vi "BioFLEX Board Switch TEENSY.vi"() -> ()   [LabVIEW 2015]
uses:
  <vilib>/DAQmx/write.llb/DAQmx Write (Digital 1D Bool 1Chan 1Samp).vi
  <vilib>/DAQmx/create/channels.llb/DAQmx Create Channel (DO-Digital Output).vi
  <vilib>/DAQmx/miscellaneous.llb/DAQmx Fill In Error Info.vi
panel:
  in  "MUX 4":T1(ring)
  in  "MUX 3":T1(ring)
  in  "MUX 2":T1(ring)
  in  "MUX 1":T1(ring)
  in  "MUX 4 Enable":bool=TRUE
  in  "MUX 3 Enable":bool=TRUE
  in  "stop":bool
  in  "MUX 1 Enable":bool=TRUE
  in  "MUX 2 Enable":bool=TRUE
  in  "POWER":bool
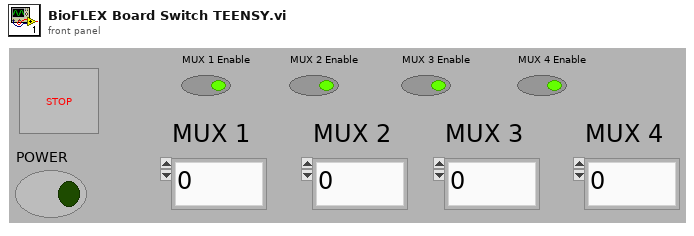
[diagram p1: front panel]
types:
  T1 = enum16{"0", "1", "2", "3", "4", "5", "6", "7", "8", "9", "10", "11", "12", "13", "14", "15", "16"}
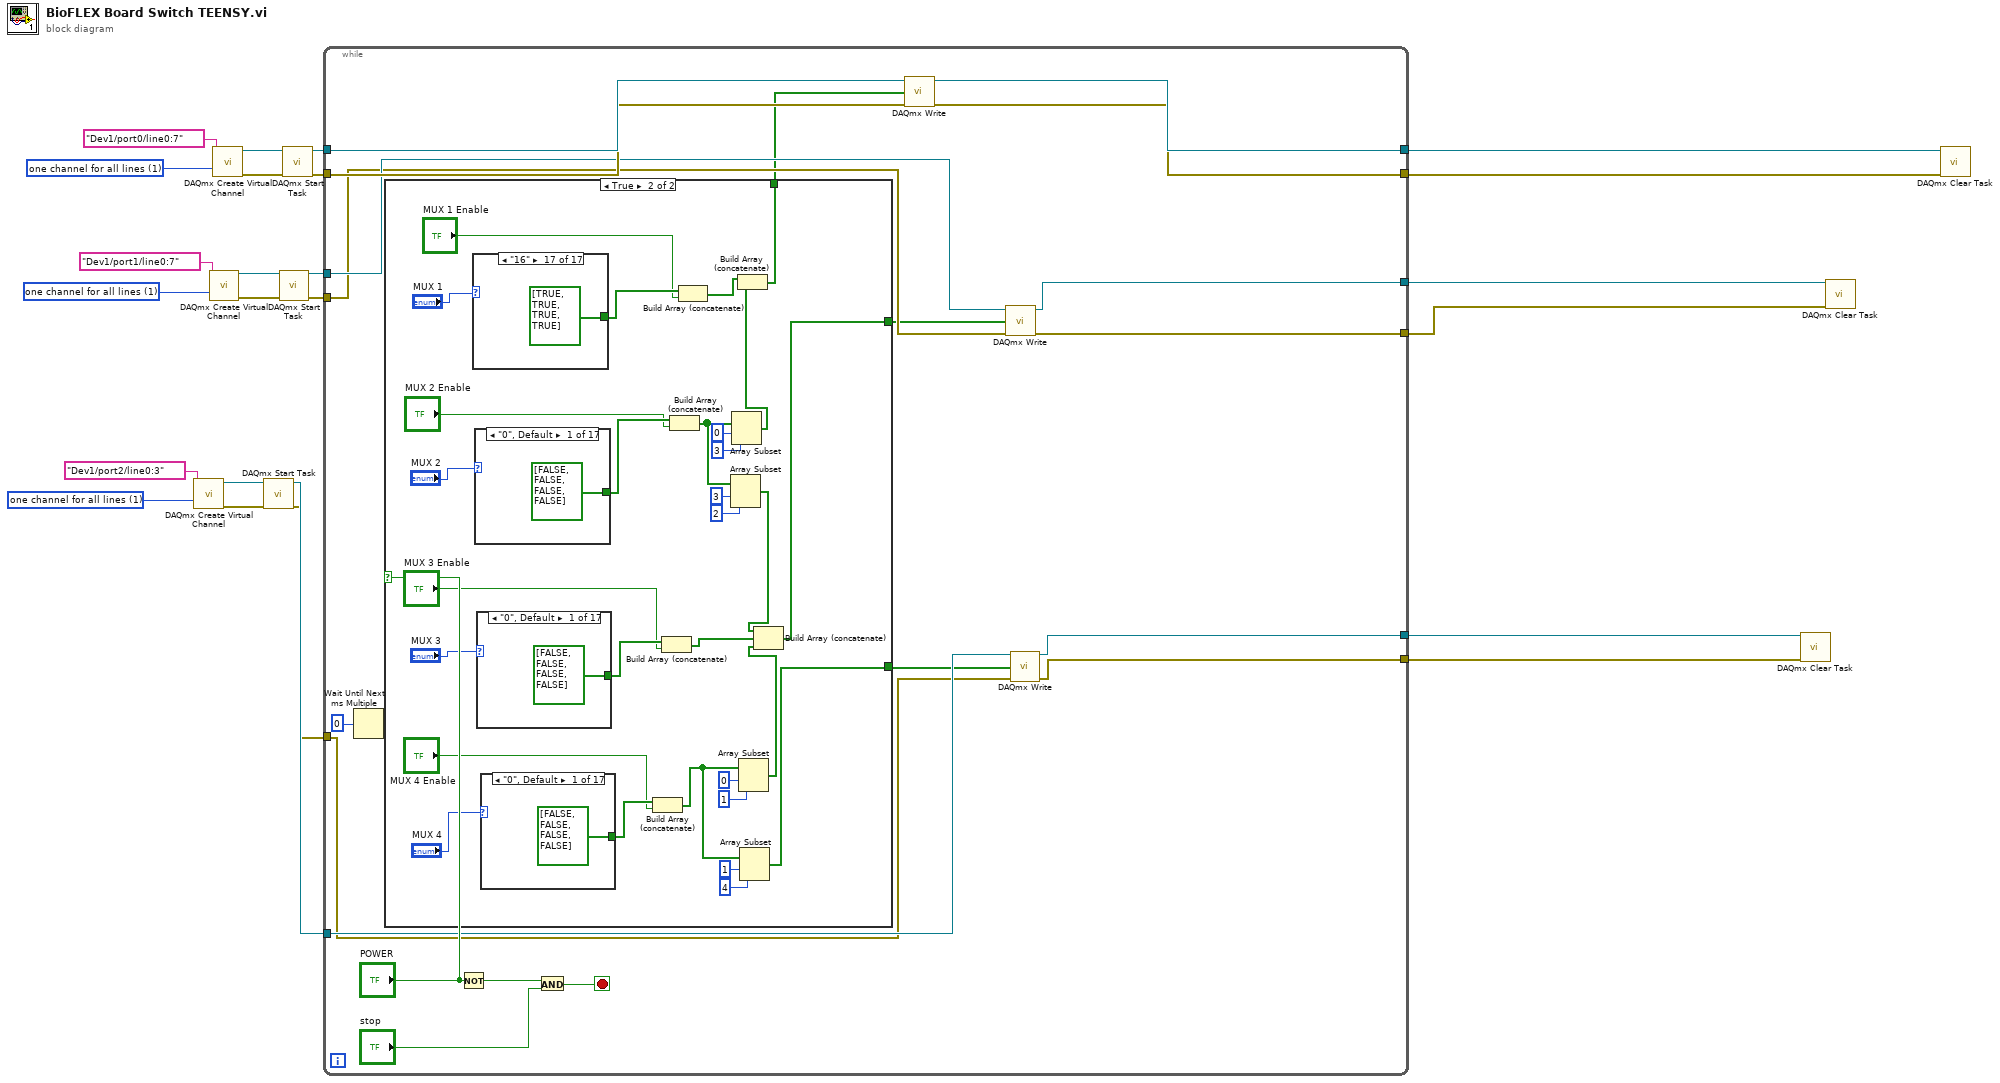
[diagram p0: block diagram]
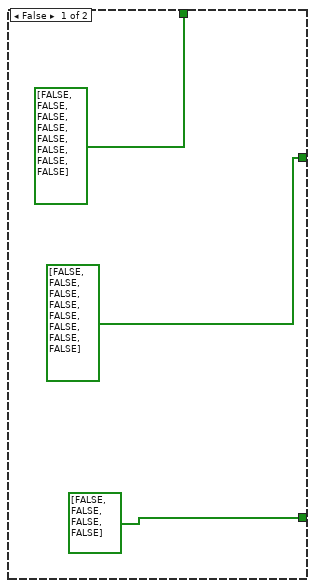
[diagram p2: hidden frame]
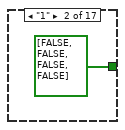
[diagram p3: hidden frame]
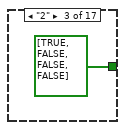
[diagram p4: hidden frame]
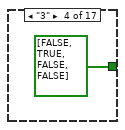
[diagram p5: hidden frame]
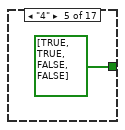
[diagram p6: hidden frame]
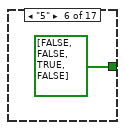
[diagram p7: hidden frame]
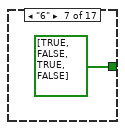
[diagram p8: hidden frame]
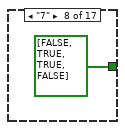
[diagram p9: hidden frame]
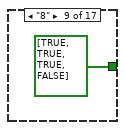
[diagram p10: hidden frame]
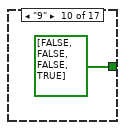
[diagram p11: hidden frame]
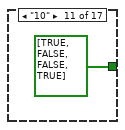
[diagram p12: hidden frame]
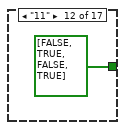
[diagram p13: hidden frame]
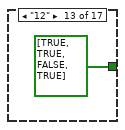
[diagram p14: hidden frame]
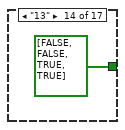
[diagram p15: hidden frame]
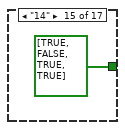
[diagram p16: hidden frame]
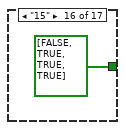
[diagram p17: hidden frame]
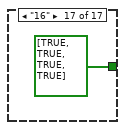
[diagram p18: hidden frame]
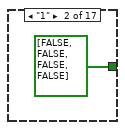
[diagram p19: hidden frame]
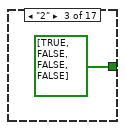
[diagram p20: hidden frame]
diagram:
  w12 = 1 items=["one channel for each line", "one channel for all lines"] ("line grouping")
  w16 = 1 items=["one channel for each line", "one channel for all lines"] ("line grouping")
  w24 = 1 items=["one channel for each line", "one channel for all lines"] ("line grouping")
  n1 = call-poly <vilib>:"DAQmx Create Virtual Channel.vi"("lines"=tag "Dev1/port2/line0:3", "line grouping"=w12) -> ("task out"=w10:refnum<k21>, "error out"=w11:errorcluster)  [unwired: 12 in]
  n2 = call-poly <vilib>:"DAQmx Create Virtual Channel.vi"("lines"=tag "Dev1/port1/line0:7", "line grouping"=w16) -> ("task out"=w14:refnum<k21>, "error out"=w15:errorcluster)  [unwired: 12 in]
  n3 = call-poly <vilib>:"DAQmx Create Virtual Channel.vi"("lines"=tag "Dev1/port0/line0:7", "line grouping"=w24) -> ("task out"=w22:refnum<k21>, "error out"=w23:errorcluster)  [unwired: 12 in]
  n4 = call <vilib>:"DAQmx Start Task.vi"("task/channels in"=w10, "error in"=w11) -> ("task out"=w2:refnum<k21>, "error out"=w1:errorcluster)  [unwired: 12 in]
  n5 = call <vilib>:"DAQmx Start Task.vi"("task/channels in"=w14, "error in"=w15) -> ("task out"=w4:refnum<k21>, "error out"=w3:errorcluster)  [unwired: 12 in]
  n6 = call <vilib>:"DAQmx Start Task.vi"("task/channels in"=w22, "error in"=w23) -> ("task out"=w21:refnum<k21>, "error out"=w20:errorcluster)  [unwired: 12 in]
  n7 = while {
    tunnel: w21 -> [w44]
    tunnel: w20 -> [w43]
    tunnel: [w42] -> w19
    tunnel: [w41] -> w18
    tunnel: [w35] -> w8
    tunnel: [w34] -> w7
    tunnel: [w33] -> w6
    tunnel: [w32] -> w5
    tunnel: w4 -> [w31]
    tunnel: w3 -> [w30]
    tunnel: w2 -> [w29]
    tunnel: w1 -> [w28]
    stop <- w37 stop-if-true
    n8 = Wait Until Next ms Multiple(millisecond multiple=u32 0 ("milliseconds to wait")) -> ()  [unwired: 1 out]
    n9 = case shown="True" "POWER" {
      tunnel: [bool[] [FALSE, FALSE, FALSE, FALSE, FALSE, FALSE, FALSE, FALSE] w62] -> w27
      tunnel: [bool[] [FALSE, FALSE, FALSE, FALSE, FALSE, FALSE, FALSE, FALSE] w55] -> w26
      tunnel: [bool[] [FALSE, FALSE, FALSE, FALSE] w48] -> w25
      frame False {
      }
      frame True {
        n10 = case shown="\"16\"" "MUX 1" {
          tunnel: [bool[] [FALSE, FALSE, FALSE, FALSE] bool[] [FALSE, FALSE, FALSE, FALSE] bool[] [TRUE, FALSE, FALSE, FALSE] bool[] [FALSE, TRUE, FALSE, FALSE] bool[] [TRUE, TRUE, FALSE, FALSE] bool[] [FALSE, FALSE, TRUE, FALSE] bool[] [TRUE, FALSE, TRUE, FALSE] bool[] [FALSE, TRUE, TRUE, FALSE] bool[] [TRUE, TRUE, TRUE, FALSE] bool[] [FALSE, FALSE, FALSE, TRUE] bool[] [TRUE, FALSE, FALSE, TRUE] bool[] [FALSE, TRUE, FALSE, TRUE] bool[] [TRUE, TRUE, FALSE, TRUE] bool[] [FALSE, FALSE, TRUE, TRUE] bool[] [TRUE, FALSE, TRUE, TRUE] bool[] [FALSE, TRUE, TRUE, TRUE] bool[] [TRUE, TRUE, TRUE, TRUE]] -> w77
          frame "0", Default {
          }
          frame "1" {
          }
          frame "2" {
          }
          frame "3" {
          }
          frame "4" {
          }
          frame "5" {
          }
          frame "6" {
          }
          frame "7" {
          }
          frame "8" {
          }
          frame "9" {
          }
          frame "10" {
          }
          frame "11" {
          }
          frame "12" {
          }
          frame "13" {
          }
          frame "14" {
          }
          frame "15" {
          }
          frame "16" {
          }
        }
        n11 = case shown="\"0\", Default" "MUX 2" {
          tunnel: [bool[] [FALSE, FALSE, FALSE, FALSE] bool[] [FALSE, FALSE, FALSE, FALSE] bool[] [TRUE, FALSE, FALSE, FALSE] bool[] [FALSE, TRUE, FALSE, FALSE] bool[] [TRUE, TRUE, FALSE, FALSE] bool[] [FALSE, FALSE, TRUE, FALSE] bool[] [TRUE, FALSE, TRUE, FALSE] bool[] [FALSE, TRUE, TRUE, FALSE] bool[] [TRUE, TRUE, TRUE, FALSE] bool[] [FALSE, FALSE, FALSE, TRUE] bool[] [TRUE, FALSE, FALSE, TRUE] bool[] [FALSE, TRUE, FALSE, TRUE] bool[] [TRUE, TRUE, FALSE, TRUE] bool[] [FALSE, FALSE, TRUE, TRUE] bool[] [TRUE, FALSE, TRUE, TRUE] bool[] [FALSE, TRUE, TRUE, TRUE] bool[] [TRUE, TRUE, TRUE, TRUE]] -> w75
          frame "0", Default {
          }
          frame "1" {
          }
          frame "2" {
          }
          frame "3" {
          }
          frame "4" {
          }
          frame "5" {
          }
          frame "6" {
          }
          frame "7" {
          }
          frame "8" {
          }
          frame "9" {
          }
          frame "10" {
          }
          frame "11" {
          }
          frame "12" {
          }
          frame "13" {
          }
          frame "14" {
          }
          frame "15" {
          }
          frame "16" {
          }
        }
        n12 = case shown="\"0\", Default" "MUX 3" {
          tunnel: [bool[] [FALSE, FALSE, FALSE, FALSE] bool[] [FALSE, FALSE, FALSE, FALSE] bool[] [TRUE, FALSE, FALSE, FALSE] bool[] [FALSE, TRUE, FALSE, FALSE] bool[] [TRUE, TRUE, FALSE, FALSE] bool[] [FALSE, FALSE, TRUE, FALSE] bool[] [TRUE, FALSE, TRUE, FALSE] bool[] [FALSE, TRUE, TRUE, FALSE] bool[] [TRUE, TRUE, TRUE, FALSE] bool[] [FALSE, FALSE, FALSE, TRUE] bool[] [TRUE, FALSE, FALSE, TRUE] bool[] [FALSE, TRUE, FALSE, TRUE] bool[] [TRUE, TRUE, FALSE, TRUE] bool[] [FALSE, FALSE, TRUE, TRUE] bool[] [TRUE, FALSE, TRUE, TRUE] bool[] [FALSE, TRUE, TRUE, TRUE] bool[] [TRUE, TRUE, TRUE, TRUE]] -> w73
          frame "0", Default {
          }
          frame "1" {
          }
          frame "2" {
          }
          frame "3" {
          }
          frame "4" {
          }
          frame "5" {
          }
          frame "6" {
          }
          frame "7" {
          }
          frame "8" {
          }
          frame "9" {
          }
          frame "10" {
          }
          frame "11" {
          }
          frame "12" {
          }
          frame "13" {
          }
          frame "14" {
          }
          frame "15" {
          }
          frame "16" {
          }
        }
        n13 = case shown="\"0\", Default" "MUX 4" {
          tunnel: [bool[] [FALSE, FALSE, FALSE, FALSE] bool[] [FALSE, FALSE, FALSE, FALSE] bool[] [TRUE, FALSE, FALSE, FALSE] bool[] [FALSE, TRUE, FALSE, FALSE] bool[] [TRUE, TRUE, FALSE, FALSE] bool[] [FALSE, FALSE, TRUE, FALSE] bool[] [TRUE, FALSE, TRUE, FALSE] bool[] [FALSE, TRUE, TRUE, FALSE] bool[] [TRUE, TRUE, TRUE, FALSE] bool[] [FALSE, FALSE, FALSE, TRUE] bool[] [TRUE, FALSE, FALSE, TRUE] bool[] [FALSE, TRUE, FALSE, TRUE] bool[] [TRUE, TRUE, FALSE, TRUE] bool[] [FALSE, FALSE, TRUE, TRUE] bool[] [TRUE, FALSE, TRUE, TRUE] bool[] [FALSE, TRUE, TRUE, TRUE] bool[] [TRUE, TRUE, TRUE, TRUE]] -> w71
          frame "0", Default {
          }
          frame "1" {
          }
          frame "2" {
          }
          frame "3" {
          }
          frame "4" {
          }
          frame "5" {
          }
          frame "6" {
          }
          frame "7" {
          }
          frame "8" {
          }
          frame "9" {
          }
          frame "10" {
          }
          frame "11" {
          }
          frame "12" {
          }
          frame "13" {
          }
          frame "14" {
          }
          frame "15" {
          }
          frame "16" {
          }
        }
        n14 = Build Array (concatenate)(w71, "MUX 4 Enable") -> (w51:bool[])
        n15 = Build Array (concatenate)(w73, "MUX 3 Enable") -> (w56:bool[])
        n16 = Build Array (concatenate)(w75, "MUX 2 Enable") -> (w60:bool[])
        n17 = Build Array (concatenate)(w77, "MUX 1 Enable") -> (w64:bool[])
        n18 = Array Subset(array=w60, index=3, length=2) -> (w57:bool[])
        n19 = Array Subset(array=w60, index=0, length=3) -> (w63:bool[])
        n20 = Build Array (concatenate)(w64, w63) -> (w62:bool[])
        n21 = Array Subset(array=w51, index=0, length=1) -> (w52:bool[])
        n22 = Array Subset(array=w51, index=1, length=4) -> (w48:bool[])
        n23 = Build Array (concatenate)(w57, w56, w52) -> (w55:bool[])
      }
    }
    n24 = Not(x="POWER") -> (.not. x?=w39:bool)
    n25 = And(x=w39, y="stop") -> (x .and. y?=w37:bool)
    n26 = call-poly <vilib>:"DAQmx Write.vi"("task/channels in"=w44, "data"=w27, "error in"=w43) -> ("task out"=w42:refnum<k21>, "error out"=w41:errorcluster)  [unwired: 10 in, 1 out]
    n27 = call-poly <vilib>:"DAQmx Write.vi"("task/channels in"=w31, "data"=w26, "error in"=w30) -> ("task out"=w35:refnum<k21>, "error out"=w33:errorcluster)  [unwired: 10 in, 1 out]
    n28 = call-poly <vilib>:"DAQmx Write.vi"("task/channels in"=w29, "data"=w25, "error in"=w28) -> ("task out"=w34:refnum<k21>, "error out"=w32:errorcluster)  [unwired: 10 in, 1 out]
  }
  n29 = call <vilib>:"DAQmx Clear Task.vi"("task in"=w7, "error in"=w5) -> ()  [unwired: 13 in, 1 out]
  n30 = call <vilib>:"DAQmx Clear Task.vi"("task in"=w8, "error in"=w6) -> ()  [unwired: 13 in, 1 out]
  n31 = call <vilib>:"DAQmx Clear Task.vi"("task in"=w19, "error in"=w18) -> ()  [unwired: 13 in, 1 out]
